vi "returns status string subvi$.vi"(0 "VISA resource name 2":refnum<visa-resource-name>="GPIB0::12::INSTR", 1 "error in (no error) 2":errorcluster) -> (2 "VISA resource name out 2":refnum<visa-resource-name>, 3 "read buffer 2":string, 4 "error out 2":errorcluster)   [LabVIEW 2009]
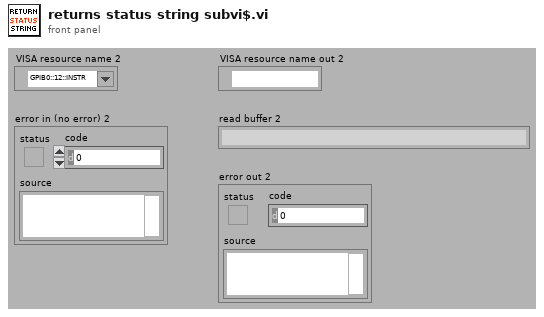
[diagram p1: front panel]
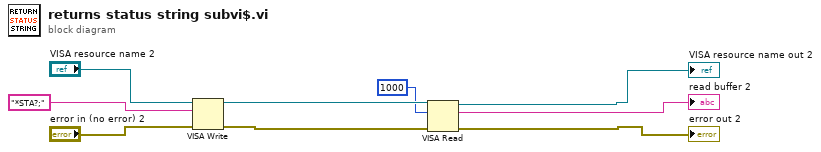
[diagram p0: block diagram]
diagram:
  n1 = VISA Write(VISA resource name="VISA resource name 2", write buffer="*STA?;" ("write buffer 2"), error in (no error)="error in (no error) 2") -> (VISA resource name out=w7:refnum<visa-resource-name>, error out=w8:errorcluster)  [unwired: 1 out]
  n2 = VISA Read(VISA resource name=w7, byte count=u32 1000 ("bytes to read (1000) 2"), error in (no error)=w8) -> (VISA resource name out=→"VISA resource name out 2":refnum<visa-resource-name>, read buffer=→"read buffer 2":string, error out=→"error out 2":errorcluster)  [unwired: 1 out]
